vi "Data_Swiss Roll.vi"(6 "seed":i32=-1, 9 "# of classes":i32=6, 11 "# of points":i32=1024) -> (1 "class":i32[](array[numeric]), 3 "Data":dbl[][](array[numeric]))   [LabVIEW 2009]
uses:
  <vilib>/Analysis/NI_AALBase.lvlib
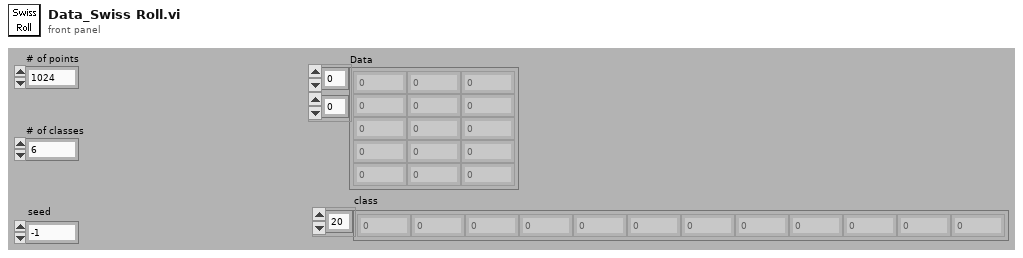
[diagram p1: front panel]
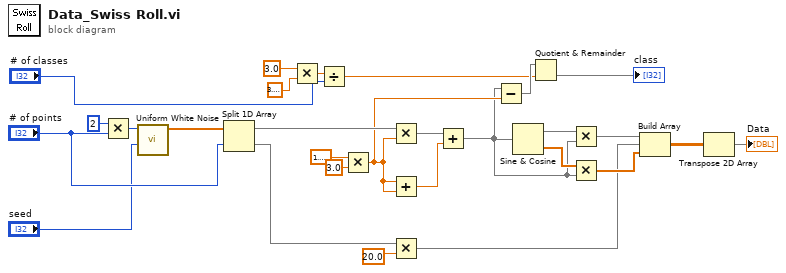
[diagram p0: block diagram]
diagram:
  n1 = Multiply(x=2, y="# of points") -> (x*y=w18:i32)
  n2 = call <vilib>:"Uniform White Noise.vi"("seed"="seed", "samples"=w18) -> ("uniform white noise"=w16:dbl[])  [unwired: 8 in, 1 out]
  n3 = Split 1D Array(array=w16, index="# of points") -> (first subarray=w15:dbl[], second subarray=w13:dbl[])
  n4 = Multiply(x=3.0, y=3.141592653589793) -> (x*y=w7:dbl)
  n5 = Divide(x=w7, y="# of classes") -> (x/y=w2:dbl)
  n6 = Multiply(x=1.5707963267948966, y=3.0) -> (x*y=w5:dbl)
  n7 = Multiply(x=w15, y=w5) -> (x*y=w20:dbl[])
  n8 = Add(x=w5, y=w5) -> (x+y=w19:dbl)
  n9 = Multiply(x=w13, y=20.0) -> (x*y=w12:dbl[])
  n10 = Add(x=w20, y=w19) -> (x+y=w4:dbl[])
  n11 = Subtract(x=w4, y=w5) -> (x-y=w3:dbl[])
  n12 = Sine & Cosine(0:w4) -> (1:w26:dbl[], 2:w25:dbl[])
  n13 = Quotient & Remainder(x=w3, y=w2) -> (floor(x/y)=→"class":dbl[])  [unwired: 1 out]
  n14 = Multiply(x=w26, y=w4) -> (x*y=w24:dbl[])
  n15 = Multiply(x=w25, y=w4) -> (x*y=w21:dbl[])
  n16 = Build Array(w24, w12, w21) -> (w23:dbl[][])
  n17 = Transpose 2D Array(2D array=w23) -> (transposed array=→"Data":dbl[][])
